vi "Queue_log_event.vi"(7 "Subsystem name in":string, 9 "Event or Warning":T1, 10 "Event discription in":string) -> (3 "queue out":refnum<queue>)   [LabVIEW 2017, in "labview-standard-library.lvlib"]
uses:
  labview-standard-library.lvlib
  Event_type_selecter.ctl
  Time&Event_cluster.ctl
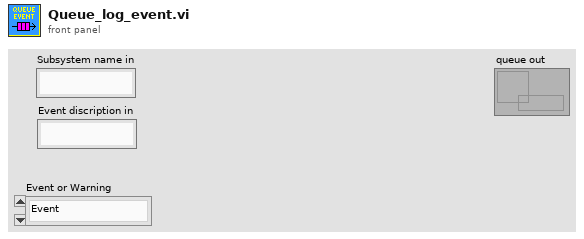
[diagram p1: front panel]
types:
  T1 = typedef "labview-standard-library.lvlib/Event_type_selecter.ctl" = enum16{"Event", "Warning", "Write events"}
  T2 = typedef "labview-standard-library.lvlib/Time&Event_cluster.ctl" = cluster{"Time in seconds":dbl, "Event text":string}
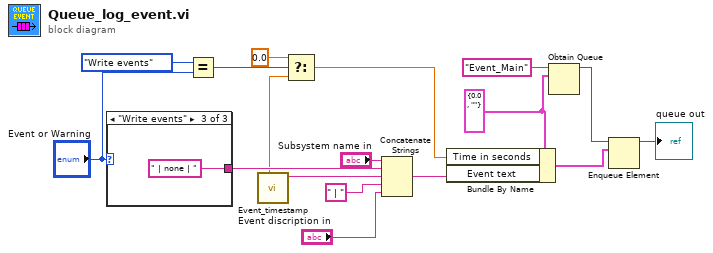
[diagram p0: block diagram]
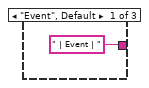
[diagram p2: hidden frame]
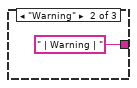
[diagram p3: hidden frame]
diagram:
  w7 = T2 {"Time in seconds"=0.0, "Event text"=""} ("Cluster")
  n1 = case shown="\"Write events\"" "Event or Warning" {
    tunnel: [" | Event | " " | Warning | " " | none | "] -> w13
    frame "Event", Default {
    }
    frame "Warning" {
    }
    frame "Write events" {
    }
  }
  n2 = Equal?(x=Event_type_selecter."Write events", y="Event or Warning") -> (x = y?=w3:bool)
  n3 = call "Event_timestamp.vi"() -> ("date/time string"=w17:string, "Raw time output"=w4:dbl)  [unwired: 10 in]
  n4 = Select(t=0.0, s=w3, f=w4) -> (s? t:f=w1:dbl)
  n5 = Concatenate Strings("Subsystem name in", w13, w17, " | ", "Event discription in") -> (w12:string)
  n6 = Bundle By Name(cluster=w7, "Time in seconds"=w1, "Event text"=w12) -> (w11:T2)
  n7 = Obtain Queue(name (unnamed)="Event_Main", element data type=w7) -> (queue out=w8:refnum<queue>)  [unwired: 3 in, 2 out]
  n8 = Enqueue Element(queue=w8, element=w11) -> (queue out=→"queue out":refnum<queue>)  [unwired: 2 in, 2 out]
